vi "MTMount_putSample_Azimuth.vi"(8 "error in (no error)":errorcluster, 11 "Azimuth_Ctl":T1) -> (0 "error out":errorcluster, 2 "function return":i32, 3 "Azimuth_Ctl out":T1)   [LabVIEW 2018, in "SALLV_MTMount.lvlib"]
doc: "int MTMount_shm_putSample_AzimuthLV(MTMount_AzimuthLV *Azimuth_Ctl );"
uses:
  SALLV_MTMount.lvlib
  DataTypes/Azimuth.ctl
  SALLV_MTMount.so
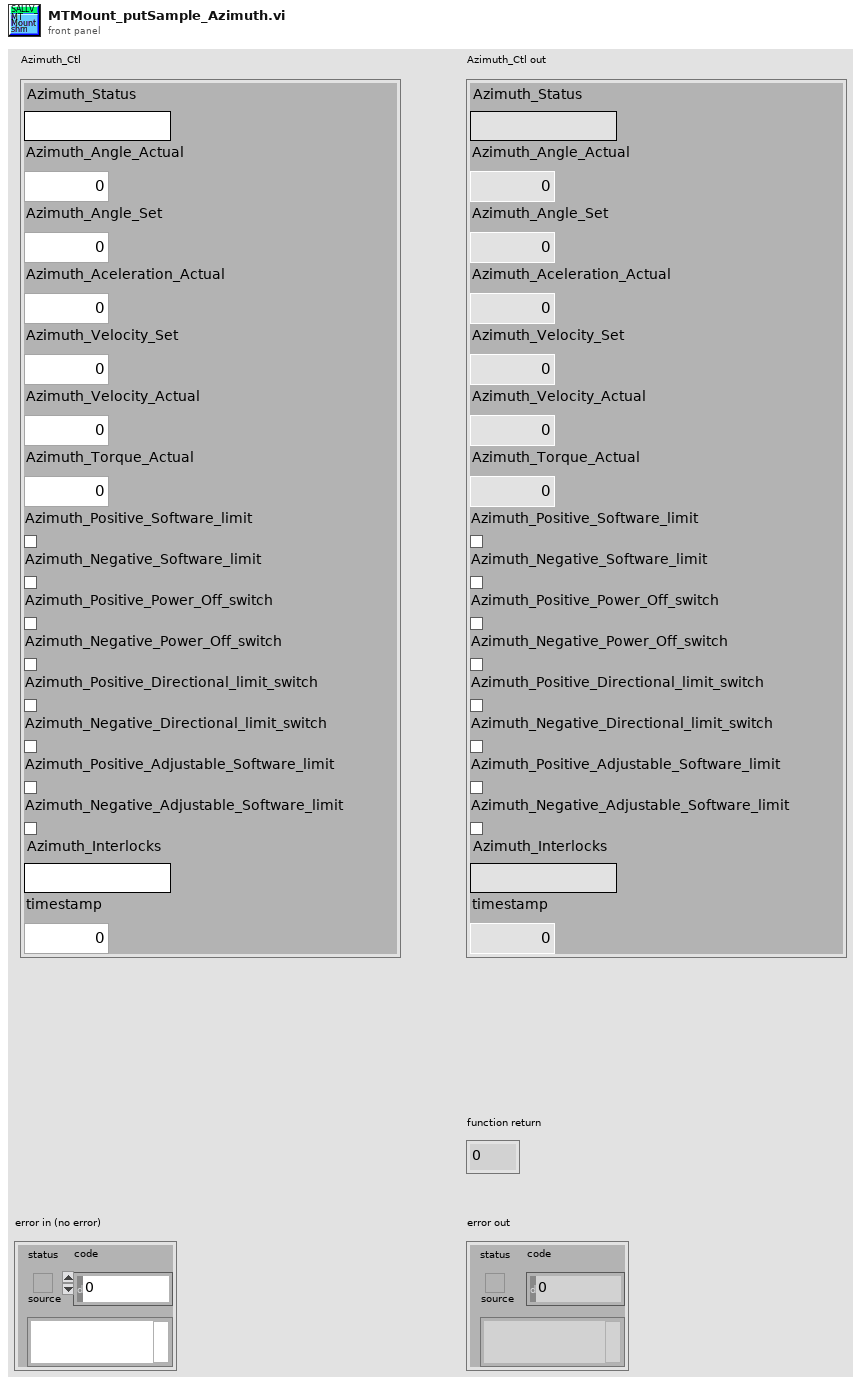
[diagram p1: front panel]
types:
  T1 = typedef "SALLV_MTMount.lvlib/Azimuth.ctl" = cluster{"Azimuth_Status":string, "Azimuth_Angle_Actual":dbl, "Azimuth_Angle_Set":dbl, "Azimuth_Aceleration_Actual":dbl, "Azimuth_Velocity_Set":dbl, "Azimuth_Velocity_Actual":dbl, "Azimuth_Torque_Actual":dbl, "Azimuth_Positive_Software_limit":bool, "Azimuth_Negative_Software_limit":bool, "Azimuth_Positive_Power_Off_switch":bool, "Azimuth_Negative_Power_Off_switch":bool, "Azimuth_Positive_Directional_limit_switch":bool, "Azimuth_Negative_Directional_limit_switch":bool, "Azimuth_Positive_Adjustable_Software_limit":bool, "Azimuth_Negative_Adjustable_Software_limit":bool, "Azimuth_Interlocks":string, "timestamp":dbl}
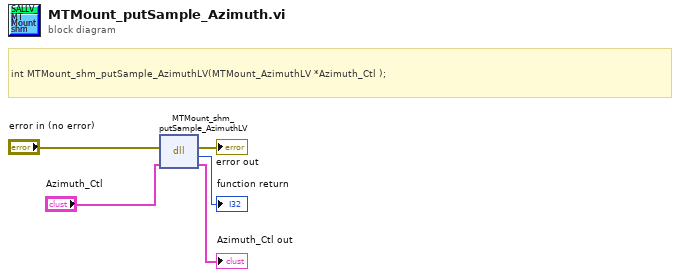
[diagram p0: block diagram]
diagram:
  # "int MTMount_shm_putSample_AzimuthLV(MTMount_AzimuthLV *Azimuth_Ctl );"
  n1 = dll-call lib="home/ttsai/Document/salApiMTMount/SALLV_MTMount/SALLV_MTMount.*" fn="MTMount_shm_putSample_AzimuthLV"(error in="error in (no error)", "Azimuth_Ctl"="Azimuth_Ctl") -> (error out=→"error out":errorcluster, →"function return":i32, "Azimuth_Ctl"=→"Azimuth_Ctl out":T1)  [unwired: 2 in, 1 out]
